vi "Do.vi"(8 "error in (no error)":errorcluster, 10 "Actor in":refnum<class "Actor.lvclass">, 11 "Log Event Msg":refnum<class "Log Event Msg.lvclass">) -> (0 "error out":errorcluster, 2 "Actor out":refnum<class "Actor.lvclass">)   [LabVIEW 2014, in "MWWL Verification.lvlib" / "Log Event Msg.lvclass"]
uses:
  Log Event Msg.lvclass
  <vilib>/ActorFramework/Actor/Actor.lvclass
  MWWL Verification/MWWL Verification.lvclass
  Log Event Msg.lvclass/Log Event Msg.ctl
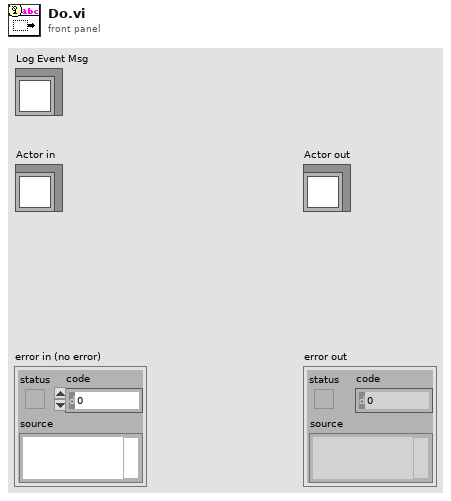
[diagram p1: front panel]
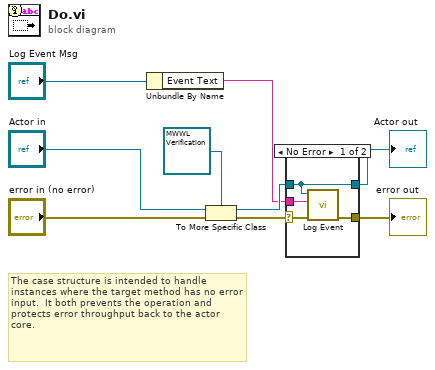
[diagram p0: block diagram]
diagram:
  # "The case structure is intended to handle instances where the target method has no error input.  It both prevents the operation and protects error throughput back to the actor core."
  n1 = Unbundle By Name("Log Event Msg") -> ("Event Text"=w2:string)
  n2 = To More Specific Class(target class=refnum<class "MWWL Verification.lvclass"> refnum ("Actor in"), reference="Actor in", error in="error in (no error)") -> (specific class reference=w9:refnum<class "MWWL Verification.lvclass">, error out=w5:errorcluster)
  n3 = case shown="No Error" w5 {
    selector: w5 -> [w12 w15]
    tunnel: w9 -> [w10 w14]
    tunnel: [w13 w15] -> w4
    tunnel: [w10 w14] -> w3
    tunnel: w2 -> [w11 _]
    frame No Error {
      n4 = call "Log Event.vi"("error in (no error)"=w12, "Event Text"=w11, "MWWL Verification in"=w10) -> ("error out"=w13:errorcluster)  [unwired: 8 in]
    }
    frame Error {
    }
  }
  "error out" <- w4
  "Actor out" <- w3
